vi "init_input_channel.vi"(8 "error in (no error)":errorcluster, 9 "samples per channel":i32=503, 10 "rate":dbl=1000.0 format="%#_13g", 11 "input channel":tag) -> (0 "error out":errorcluster, 3 "task out":refnum<k21>)   [LabVIEW 2015]
uses:
  <vilib>/DAQmx/create/channels.llb/DAQmx Create Channel (AI-Voltage-Basic).vi
  <vilib>/DAQmx/configure/timing.llb/DAQmx Timing (Sample Clock).vi
  <resource>/objmgr/daqmx.rc
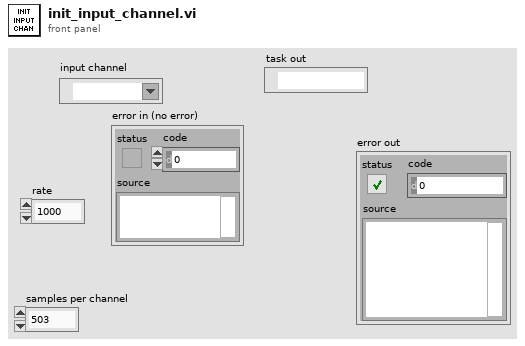
[diagram p1: front panel]
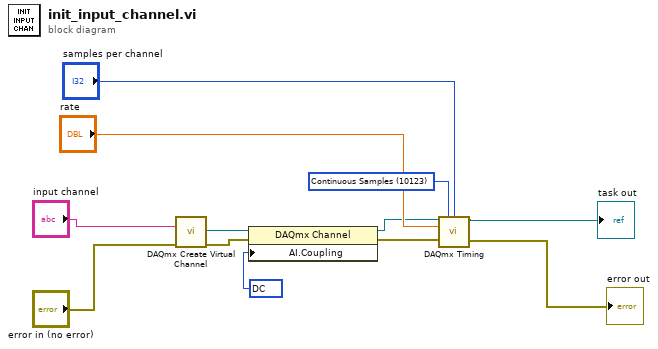
[diagram p0: block diagram]
diagram:
  w8 = 10123 items=["Finite Samples"=10178, "Continuous Samples"=10123, "Hardware Timed Single Point"=12522] ("sample mode")
  w7 = 10050 items=["AC"=10045, "DC"=10050, "GND"=10066] ("AI.Coupling")
  n1 = call-poly <vilib>:"DAQmx Create Virtual Channel.vi"("physical channels"="input channel", "error in"="error in (no error)") -> ("task out"=w5:refnum<k21>, "error out"=w6:errorcluster)  [unwired: 12 in]
  n2 = property class="DAQmx Channel"(reference=w5, error in=w6, "AI.Coupling"=w7) -> (reference out=w9:refnum<k21>, error out=w10:errorcluster)
  n3 = call-poly <vilib>:"DAQmx Timing.vi"("task/channels in"=w9, "sample mode"=w8, "samples per channel"="samples per channel", "rate"="rate", "error in"=w10) -> ("task out"=→"task out":refnum<k21>, "error out"=→"error out":errorcluster)  [unwired: 9 in]
